vi "test_library.vi"() -> ()   [LabVIEW 2018]
uses:
  type_control.ctl
panel:
  in  "file_name":string="prova.mat"
  in  "file (use dialog)":path
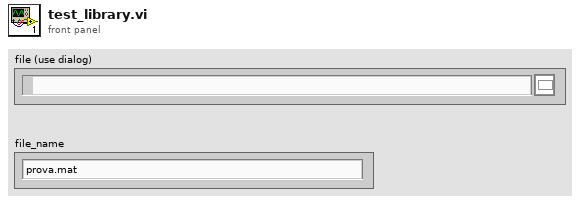
[diagram p1: front panel]
types:
  T1 = typedef "type_control.ctl" = enum16{"Int8bit_elem", "Int8bit", "Int64bit_elem", "Int64bit", "Int16bit_elem", "Double64bit_elem", "Int16bit", "Double64bit"}
  T2 = enum16{"open", "replace", "create", "open or create", "replace or create", "replace or create with confirmation"}
  T3 = typedef "MatFile_information.ctl" = cluster{"file path (use dialog)":path, "refnum file":refnum<file>, "intermediate array":cluster{"intermediate":refnum<file>, "array name dim":i32, "row":i32, "col":i32, "Content":string, "Enum":T1}[]}
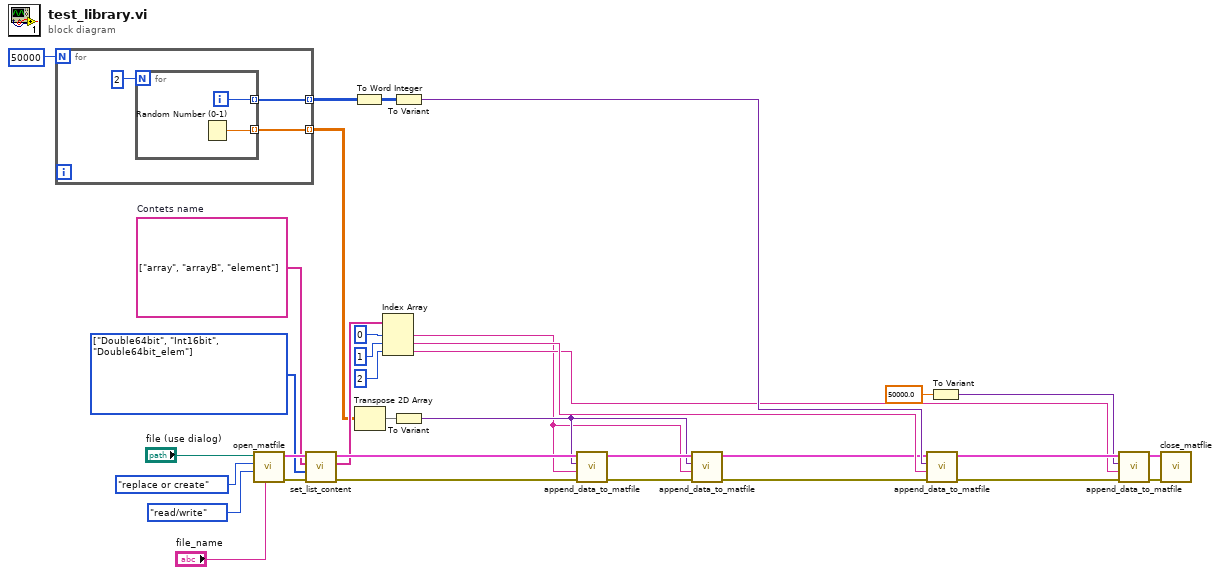
[diagram p0: block diagram]
diagram:
  w22 = T1[] [enum."Double64bit", enum."Int16bit", enum."Double64bit_elem"] items=["Int8bit_elem", "Int8bit", "Int64bit_elem", "Int64bit", "Int16bit_elem", "Double64bit_elem", "Int16bit", "Double64bit"] ("Enum")
  w26 = string[] ["array", "arrayB", "element"]  # Contets name
  n1 = for {
    N: 50000 -> [_]
    tunnel: [w36] -> w14 mode=indexing
    tunnel: [w35] -> w17 mode=indexing
    n2 = for {
      N: 2 -> [_]
      tunnel: [w39] -> w36 mode=indexing
      tunnel: [w38] -> w35 mode=indexing
      i -> [w38]
      n3 = Random Number (0-1)() -> (number: 0 to 1=w39:dbl)
    }
  }
  n4 = call "open_matfile.vi"("file_name"="file_name", "access (0:read/write)"=enum16{"read/write", "read-only", "write-only"}."read/write", "operation (0:open)"=T2."replace or create", "file path (use dialog)"="file (use dialog)") -> ("error out"=w28:errorcluster, "matFile_info"=w27:T3)  [unwired: 5 in]
  n5 = call "set_list_content.vi"("error in"=w28, "Type"=w22, "Contents"=w26, "matFile_info IN"=w27) -> ("error out"=w32:errorcluster, "Contents"=w19:string[], "matFile_info OUT"=w33:T3)  [unwired: 5 in]
  n6 = To Word Integer(number=w17) -> (16bit integer=w16:i16[][])
  n7 = Transpose 2D Array(2D array=w14) -> (transposed array=w1:dbl[][])
  n8 = Index Array(array=w19, index #1=0 ("index"), index #2=1 ("index"), index #3=2 ("index")) -> (element #1=w4:string, element #2=w34:string, element #3=w10:string)
  n9 = To Variant(anything=w16) -> (Variant=w31:variant)
  n10 = To Variant(anything=w1) -> (Variant=w5:variant)
  n11 = call "append_data_to_matfile.vi"("error in"=w32, "Content"=w4, "Variant"=w5, "matFile_info IN"=w33) -> ("error out"=w7:errorcluster, "matFile_info OUT"=w6:T3)  [unwired: 6 in]
  n12 = call "append_data_to_matfile.vi"("error in"=w7, "Content"=w4, "Variant"=w5, "matFile_info IN"=w6) -> ("error out"=w3:errorcluster, "matFile_info OUT"=w2:T3)  [unwired: 6 in]
  n13 = call "append_data_to_matfile.vi"("error in"=w3, "Content"=w34, "Variant"=w31, "matFile_info IN"=w2) -> ("error out"=w13:errorcluster, "matFile_info OUT"=w12:T3)  [unwired: 6 in]
  n14 = To Variant(anything=50000.0) -> (Variant=w11:variant)
  n15 = call "append_data_to_matfile.vi"("error in"=w13, "Content"=w10, "Variant"=w11, "matFile_info IN"=w12) -> ("error out"=w9:errorcluster, "matFile_info OUT"=w8:T3)  [unwired: 6 in]
  n16 = call "close_matflie.vi"("error in"=w9, "matFile_info IN"=w8) -> ()  [unwired: 8 in, 2 out]
